vi "Initialize Daemon.vi"(8 "error in (no error)":errorcluster, 9 "data model":refnum<class "Device Data Model.lvclass">, 10 "transmission data unit":refnum<class "Transmission Data Unit.lvclass">, 11 "network slave in":refnum<class "Network Slave.lvclass">) -> (0 "error out":errorcluster, 3 "network slave out":refnum<class "Network Slave.lvclass">)   [LabVIEW 2015, in "SubVIs.lvlib" / "Network Slave.lvclass"]
doc: "This provides an interface for the slave to launch a protocol daemon."
uses:
  <vilib>/Modbus/subvis/Protocol/Interfaces/Network Slave/Network Slave.lvclass
  <vilib>/Modbus/subvis/Transmission Data Unit (ADU)/Transmission Data Unit/Transmission Data Unit.lvclass
  <vilib>/Modbus/subvis/Data and Functions/Device Data Model/Device Data Model.lvclass
  <vilib>/Modbus/subvis/Protocol/Interfaces/Network Slave/Network Slave.lvclass/Network Slave.ctl
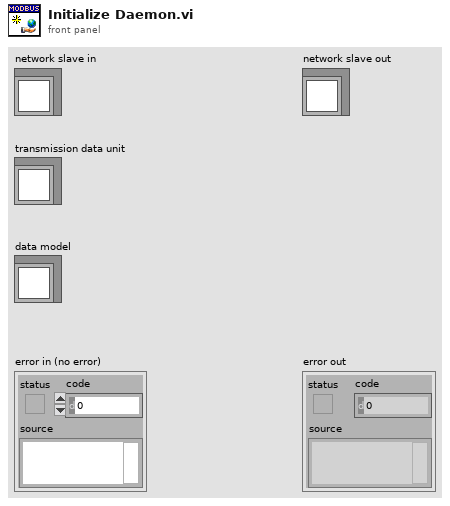
[diagram p1: front panel]
types:
  T1 = cluster{"error":errorcluster, "status":enum16{"Not Started", "Running", "Error", "Stopped"}}
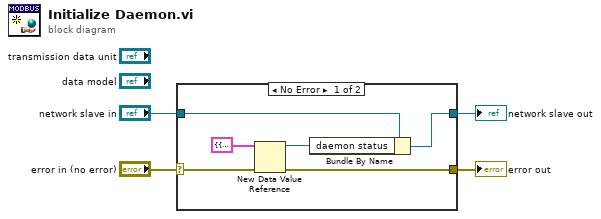
[diagram p0: block diagram]
diagram:
  n1 = case shown="No Error" "error in (no error)" {
    selector: "error in (no error)" -> [w7 w12]
    tunnel: "network slave in" -> [w10 w11]
    tunnel: [w9 w11] -> w3
    tunnel: [w6 w12] -> w1
    frame No Error {
      n2 = New Data Value Reference(data value=T1 {"error"={"status"=FALSE, "code"=0, "source"=""}, "status"=enum."Not Started"} ("Status"), error in=w7) -> (data value reference=w8:refnum<data-value>, error out=w6:errorcluster)
      n3 = Bundle By Name(cluster=w10, "daemon status"=w8) -> (w9:refnum<class "Network Slave.lvclass">)
    }
    frame Error {
    }
  }
  "error out" <- w1
  "network slave out" <- w3
